vi "Device Parameters.vi"(7 "command":T3, 8 "error in":errorcluster, 10 "Device Settings IN":T1, 11 "Device Connections IN":T2) -> (0 "error out":errorcluster, 2 "Device Settings OUT":T1, 3 "Device Connections OUT":T2)   [LabVIEW 2011]
uses:
  Device Parameters.ctl
  Controls/Device Connections.ctl
  Controls/Device Settings.ctl
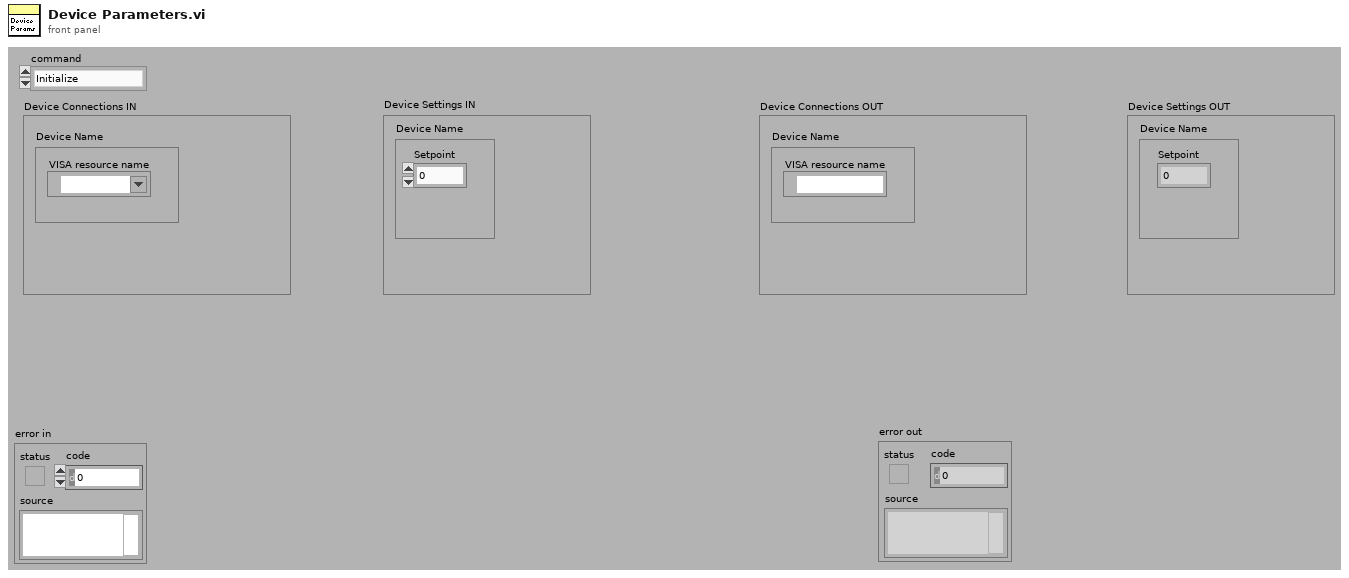
[diagram p1: front panel]
types:
  T1 = typedef "Device Settings.ctl" = cluster{"Device Name":cluster{"Setpoint":dbl}}
  T2 = typedef "Device Connections.ctl" = cluster{"Device Name":cluster{"VISA resource name":refnum<visa-resource-name>}}
  T3 = typedef "Device Parameters.ctl" = enum16{"Initialize", "Set Device Connections", "Set Device Settings", "Get Device Connections", "Get Device Settings"}
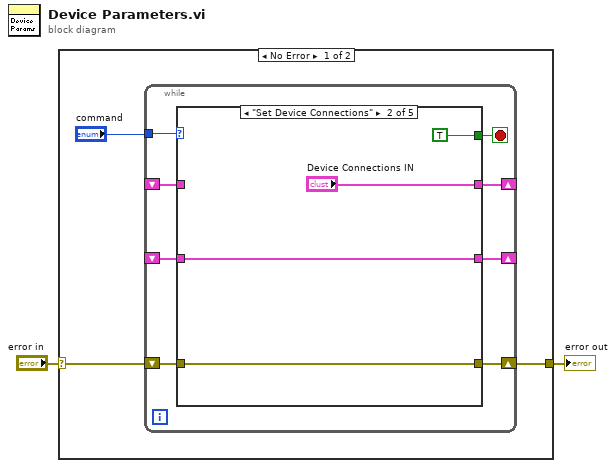
[diagram p0: block diagram]
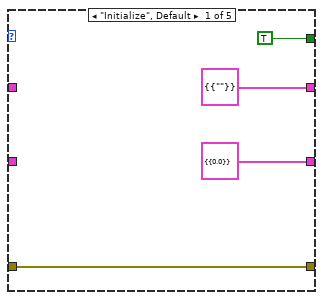
[diagram p2: hidden frame]
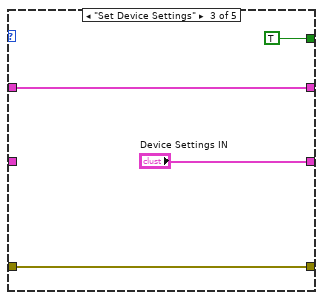
[diagram p3: hidden frame]
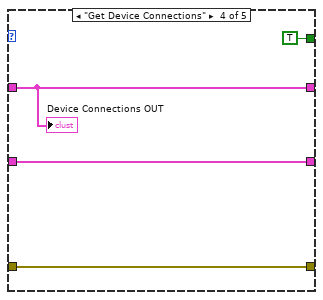
[diagram p4: hidden frame]
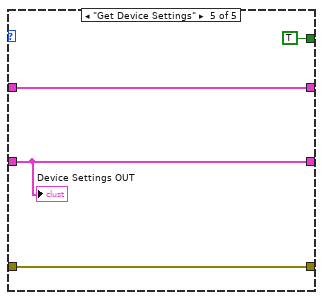
[diagram p5: hidden frame]
diagram:
  n1 = case shown="No Error" "error in" {
    selector: "error in" -> [w5 w34]
    tunnel: [w4 w34] -> w1
    frame No Error {
      n2 = while {
        shift-right: [w11] -> w4
        shift-left: w5 -> [w12]
        tunnel: "command" -> [w10]
        shift-right: [w9] -> _
        shift-left: _ -> [w6]
        shift-right: [w8] -> _
        shift-left: _ -> [w7]
        stop <- w13 stop-if-true
        n3 = case shown="\"Set Device Connections\"" w10 {
          tunnel: [TRUE TRUE TRUE TRUE TRUE] -> w13
          tunnel: w12 -> [w16 w18 w25 w26 w31]
          tunnel: [w16 w18 w25 w26 w31] -> w11
          tunnel: [T2 {"Device Name"={"VISA resource name"=""}} ("Device Connections") "Device Connections IN" w23 w28 w33] -> w9
          tunnel: [T1 {"Device Name"={"Setpoint"=0.0}} ("Device Connections") w19 "Device Settings IN" w29 w32] -> w8
          tunnel: w7 -> [_ w19 _ w29 w32]
          tunnel: w6 -> [_ _ w23 w28 w33]
          frame "Initialize", Default {
          }
          frame "Set Device Connections" {
          }
          frame "Set Device Settings" {
          }
          frame "Get Device Connections" {
            "Device Connections OUT" <- w28
          }
          frame "Get Device Settings" {
            "Device Settings OUT" <- w32
          }
        }
      }
    }
    frame Error {
    }
  }
  "error out" <- w1
